vi "11_DC Motor.vi"() -> ()   [LabVIEW 2018]
uses:
  <userlib>/KNR OS 4.0 LabVIEW Toolkit/Type Definition/Resource.ctl
  <userlib>/KNR OS 4.0 LabVIEW Toolkit/Type Definition/DC Motor Port.ctl
panel:
  in  "IP":string(combo)="172.22.11.2"
  in  "Port":T1=4 items=["DS1"=4, "DS2"=5, "DS3"=6, "DS4"=7]
  in  "Resource":T2=enum."KNRm_DDDD"
  in  "stop":bool
  in  "Enable Motor":bool
  in  "Speed (+-100%)":dbl(slide) scale=-100.0..100.0
  out "Position":i32
  out "Velocity (cts/sec)":dbl
  in  "Reverse?":bool
  in  "Reset":bool
  # "KNR/KNRm\nPort5=DS1\nPort6=DS2\nPort7=DS3\nPort8=DS4"
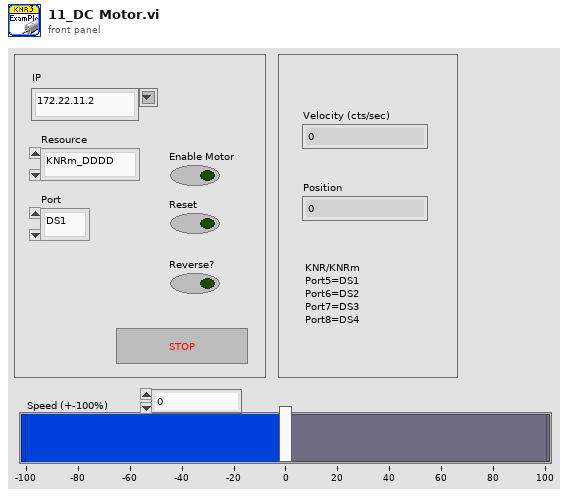
[diagram p1: front panel]
types:
  T1 = typedef "DC Motor Port.ctl" = u16
  T2 = typedef "Resource.ctl" = enum16{"KNRm_DDRC", "KNRm_DDDD", "KNRm_DDDR", "KNRm_DDDC", "KNR", "KNRm_neww"}
  T3 = typedef "KNR3 Reference.ctl" = cluster{"FPGA Session":refnum<class "FPGA Interface Base.lvclass">, "Resource":T2}
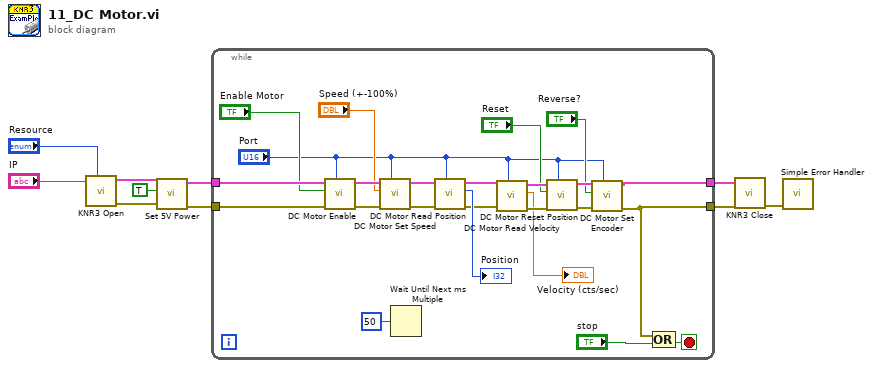
[diagram p0: block diagram]
diagram:
  n1 = call <userlib>:"KNR3 Open.vi"("Resource"="Resource", "IP"="IP") -> ("error out"=w2:errorcluster, "KNR out"=w4:T3)  [unwired: 8 in]
  n2 = call <userlib>:"Set 5V Power.vi"("error in (no error)"=w2, "5V Power(T)"=TRUE ("5V Power"), "KNR in"=w4) -> ("error out"=w8:errorcluster, "KNR out"=w9:T3)  [unwired: 7 in]
  n3 = while {
    tunnel: w9 -> [w34]
    tunnel: w8 -> [w28]
    tunnel: [w17] -> w6
    tunnel: [w18] -> w7
    stop <- w24 stop-if-true
    n4 = call <userlib>:"DC Motor Enable.vi"("Port (DS1)"="Port", "error in (no error)"=w28, "Enable Motor(F)"="Enable Motor", "KNR in"=w34) -> ("error out"=w27:errorcluster, "KNR out"=w33:T3)  [unwired: 6 in]
    n5 = call <userlib>:"DC Motor Set Speed.vi"("Port (DS1)"="Port", "error in (no error)"=w27, "Speed (+-100%)"="Speed (+-100%)", "KNR in"=w33) -> ("error out"=w26:errorcluster, "KNR out"=w32:T3)  [unwired: 6 in]
    n6 = Wait Until Next ms Multiple(millisecond multiple=u32 50) -> ()  [unwired: 1 out]
    n7 = call <userlib>:"DC Motor Read Position.vi"("Port (DS1)"="Port", "error in (no error)"=w26, "KNR in"=w32) -> ("error out"=w21:errorcluster, "Position"=→"Position":i32, "KNR out"=w22:T3)  [unwired: 6 in]
    n8 = call <userlib>:"DC Motor Read Velocity.vi"("Port (DS1)"="Port", "error in (no error)"=w21, "KNR in"=w22) -> ("error out"=w15:errorcluster, "Velocity (cts/sec)"=→"Velocity (cts/sec)":dbl, "KNR out"=w20:T3)  [unwired: 6 in]
    n9 = call <userlib>:"DC Motor Reset Position.vi"("Port (DS1)"="Port", "error in (no error)"=w15, "Reset(F)"="Reset", "KNR in"=w20) -> ("error out"=w16:errorcluster, "KNR out"=w19:T3)  [unwired: 6 in]
    n10 = call <userlib>:"DC Motor Set Encoder.vi"("Port (DS1)"="Port", "error in (no error)"=w16, "Reverse?(F)"="Reverse?", "KNR in"=w19) -> ("error out"=w17:errorcluster, "KNR out"=w18:T3)  [unwired: 6 in]
    n11 = Compound Arithmetic op=OR(w17, "stop") -> (w24:bool)
  }
  n12 = call <userlib>:"KNR3 Close.vi"("error in (no error)"=w6, "KNR in"=w7) -> ("error out"=w5:errorcluster)  [unwired: 9 in]
  n13 = call <vilib>:"Simple Error Handler.vi"("error in (no error)"=w5) -> ()  [unwired: 4 in, 5 out]
